vi "Cal-Automation module.vi"(7 "Parameter":T1, 8 "error in (no error)":errorcluster, 9 "Timed out while waiting for acknowledgement in":bool, 10 "FOR loop index":i32, 11 "Initial motor position (um)":sgl) -> (0 "error out":errorcluster, 1 "Motor timed out or errored out":bool, 2 "Cancelled":bool, 3 "Measured cal value":sgl)   [LabVIEW 2020]
uses:
  TypeDefs/Control Plane.ctl
  Globals/gl_Calibration globals.vi
panel:
  in  "Max offset (us)":i32=10 min=5 max=100
  in  "Wait before measurement (ms)":u32=500
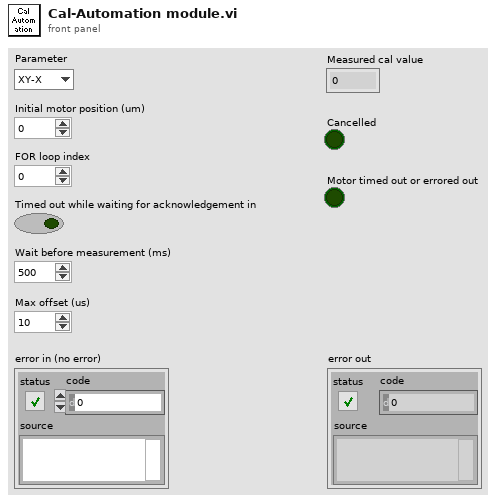
[diagram p1: front panel]
types:
  T1 = typedef "Control Plane.ctl" = enum16{"XY-X", "XY-Y", "Z"}
  T2 = typedef "AOL Z cal process refs.ctl" = cluster{"This VI":refnum<vi>, "Abort (ind)":refnum<vi>, "Next (ind)":refnum<vi>, "Cancel":refnum<vi>, "Next":refnum<vi>, "Message":refnum<vi>, "Progress":refnum<vi>}
  T3 = typedef "Cal mode.ctl" = enum16{"Automatic", "Interactive"}
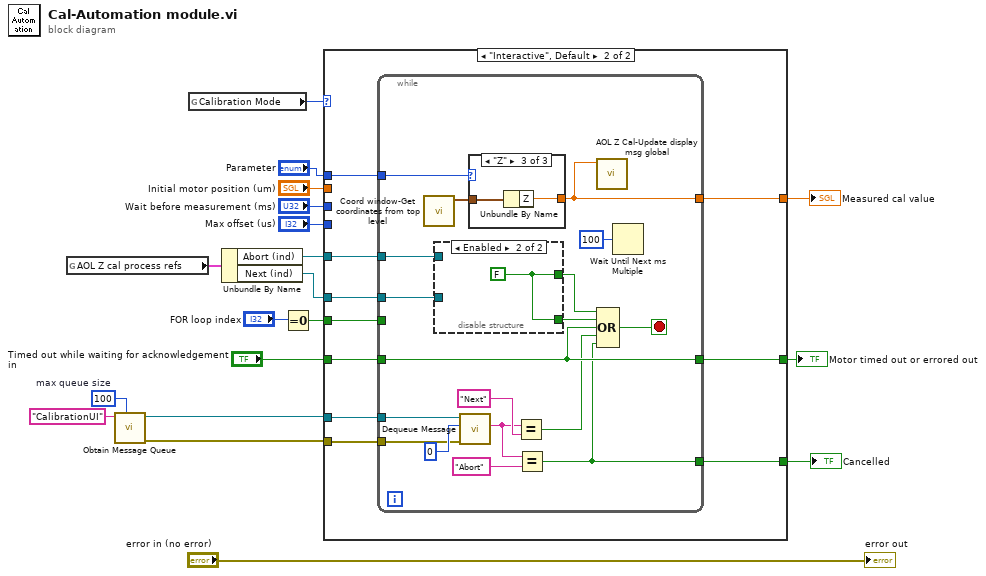
[diagram p0: block diagram]
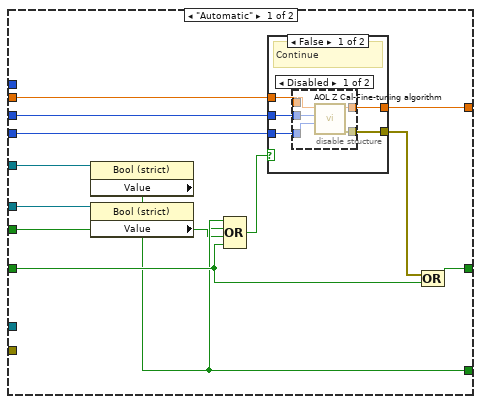
[diagram p2: hidden frame]
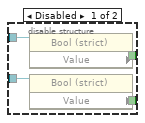
[diagram p5: hidden frame]
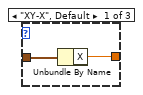
[diagram p6: hidden frame]
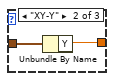
[diagram p7: hidden frame]
diagram:
  w4 = 100  # max queue size
  n1 = global read "gl_Calibration globals.vi" "AOL Z cal process refs"() -> (w13:T2)
  n2 = call "Obtain Message Queue.vi"("max queue size (-1, unlimited)"=w4, "Queue name"="CalibrationUI") -> ("error out"=w1:errorcluster, "Message Queue"=w2:refnum<queue>)  [unwired: 8 in]
  n3 = global read "gl_Calibration globals.vi" "Calibration Mode"() -> (w7:T3)
  n4 = Unbundle By Name(w13) -> ("Abort (ind)"=w18:refnum<vi>, "Next (ind)"=w19:refnum<vi>)
  n5 = Equal To 0?(x="FOR loop index") -> (x = 0?=w10:bool)
  n6 = case shown="\"Interactive\", Default" w7 {
    tunnel: w19 -> [w32 w52]
    tunnel: w18 -> [w31 w51]
    tunnel: "Initial motor position (um)" -> [w30 _]
    tunnel: [w29 w50] -> w16
    tunnel: "Timed out while waiting for acknowledgement in" -> [w28 w49]
    tunnel: [w27 w48] -> w14
    tunnel: "Wait before measurement (ms)" -> [w26 _]
    tunnel: w10 -> [w25 w47]
    tunnel: [w24 w46] -> w9
    tunnel: "Max offset (us)" -> [w23 _]
    tunnel: "Parameter" -> [_ w45]
    tunnel: w2 -> [_ w44]
    tunnel: w1 -> [_ w43]
    frame "Automatic" {
      n7 = property class="Bool (strict)"(reference=w31) -> ("Value"=w27:bool)  [unwired: 1 in, 2 out]
      n8 = property class="Bool (strict)"(reference=w32) -> ("Value"=w22:bool)  [unwired: 1 in, 2 out]
      n9 = Compound Arithmetic op=OR(w27, w22, w25, w28) -> (w21:bool)
      n10 = case shown="False" w21 {
        tunnel: w30 -> [w37 _]
        tunnel: w26 -> [w36 _]
        tunnel: [w35 _] -> w24
        tunnel: [w34 _] -> w20
        tunnel: w23 -> [w33 _]
        frame False {
          # "Continue"
          n11 = disable-structure shown="Disabled" {
            disable-tunnel: w37 -> [w42 _]
            disable-tunnel: w36 -> [w41 _]
            disable-tunnel: [w40 _] -> w35
            disable-tunnel: [w39 _] -> w34
            disable-tunnel: w33 -> [w38 _]
            frame Disabled {
              n12 = call "AOL Z Cal-Fine-tuning algorithm.vi"("Max offset (us)"=w38, "Wait before measurement (ms)"=w41, "Initial motor position (um)"=w42) -> ("error out"=w39:errorcluster, "Measured cal value"=w40:sgl)  [unwired: 7 in]
            }
            frame Enabled {
            }
          }
        }
        frame True {
          # "Abort"
        }
      }
      n13 = Compound Arithmetic op=OR(w20, w28) -> (w29:bool)
    }
    frame "Interactive", Default {
      n14 = while {
        tunnel: w52 -> [w70]
        tunnel: w51 -> [w69]
        tunnel: [w61] -> w50
        tunnel: w49 -> [w61]
        tunnel: [w53] -> w48
        tunnel: w47 -> [_]
        tunnel: [w63] -> w46
        tunnel: w45 -> [w62]
        tunnel: w44 -> [w59]
        tunnel: w43 -> [w58]
        stop <- w66 stop-if-true
        n15 = call "Coord window-Get coordinates from top level.vi"() -> ("Coordinates"=w64:cluster{"X":sgl, "Y":sgl, "Z":sgl})  [unwired: 11 in]
        n16 = disable-structure shown="Enabled" {
          disable-tunnel: w70 -> [w74 _]
          disable-tunnel: w69 -> [w73 _]
          disable-tunnel: [w72 w75] -> w68
          disable-tunnel: [w71 w75] -> w67
          frame Disabled {
            n17 = property class="Bool (strict)"(reference=w73) -> ("Value"=w72:bool)  [unwired: 1 in, 2 out]
            n18 = property class="Bool (strict)"(reference=w74) -> ("Value"=w71:bool)  [unwired: 1 in, 2 out]
          }
          frame Enabled {
            w75 = FALSE ("Value")
          }
        }
        n19 = call "Dequeue Message.vi"("Error In"=w58, "timeout in ms (-1)"=0, "Message Queue"=w59) -> ("Message"=w56:string)  [unwired: 4 in, 4 out]
        n20 = case shown="\"Z\"" w62 {
          tunnel: w64 -> [w77 w79 w81]
          tunnel: [w76 w78 w80] -> w63
          frame "XY-X", Default {
            n21 = Unbundle By Name(w77) -> ("X"=w76:sgl)
          }
          frame "XY-Y" {
            n22 = Unbundle By Name(w79) -> ("Y"=w78:sgl)
          }
          frame "Z" {
            n23 = Unbundle By Name(w81) -> ("Z"=w80:sgl)
          }
        }
        n24 = Equal?(x=w56, y="Next") -> (x = y?=w54:bool)
        n25 = Equal?(x=w56, y="Abort") -> (x = y?=w53:bool)
        n26 = call "AOL Z Cal-Update display msg global.vi"("Motor Z"=w63) -> ()  [unwired: 11 in]
        n27 = Compound Arithmetic op=OR(w68, w67, w61, w54, w53) -> (w66:bool)
        n28 = Wait Until Next ms Multiple(millisecond multiple=u32 100) -> ()  [unwired: 1 out]
      }
    }
  }
  "Motor timed out or errored out" <- w16
  "Cancelled" <- w14
  "Measured cal value" <- w9
  "error out" <- "error in (no error)"
